vi "HandleObservationSync.vi"(8 "error in (no error)":errorcluster, 11 "S4GUI in":refnum<class "S4GUI.lvclass">) -> (0 "error out":errorcluster, 3 "S4GUI out":refnum<class "S4GUI.lvclass">)   [LabVIEW 2018, in "S4GUI.lvclass"] (continued)
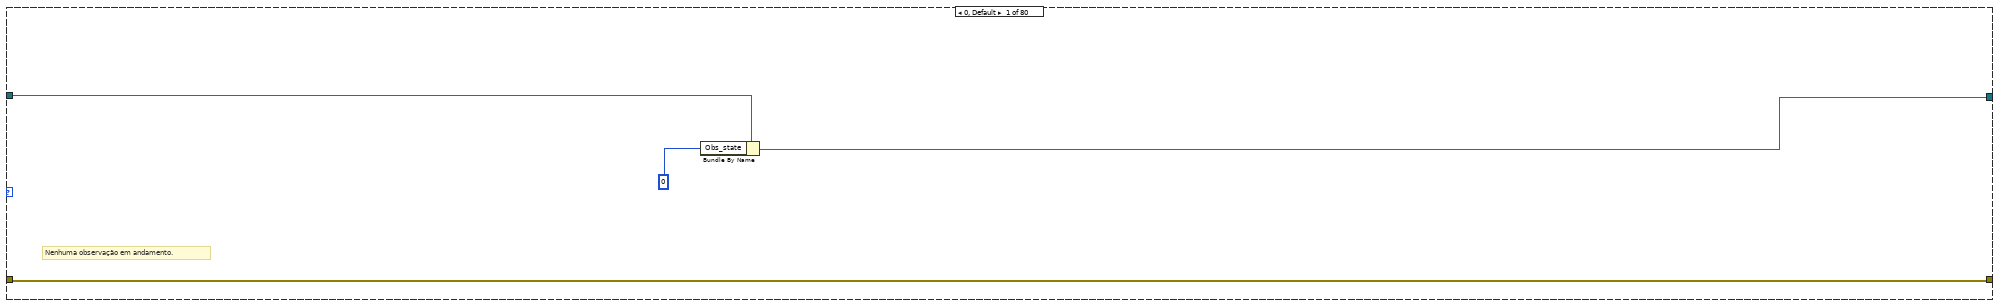
[diagram p2: hidden frame]
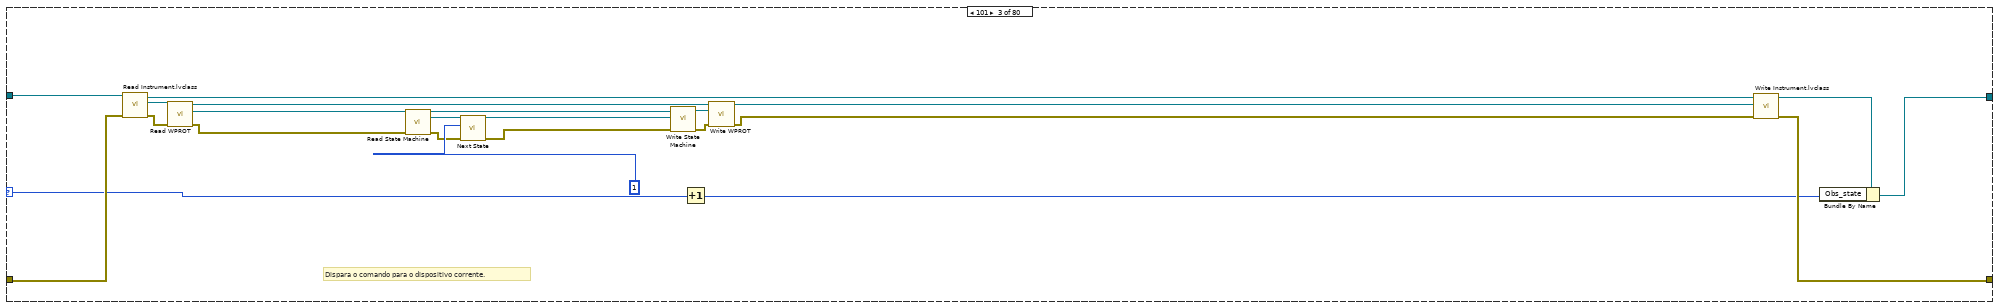
[diagram p4: hidden frame]
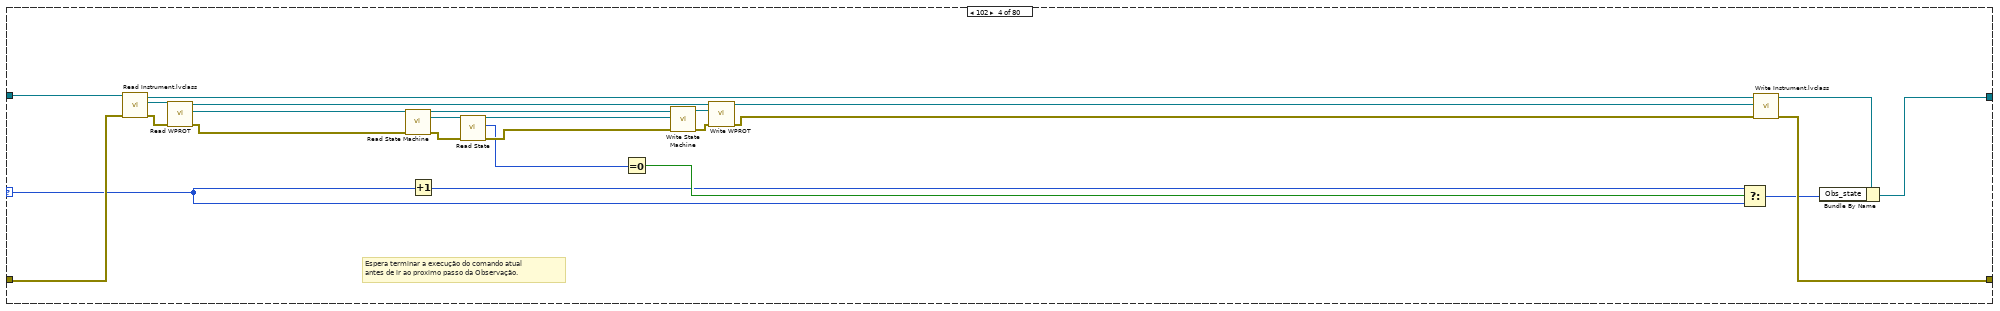
[diagram p5: hidden frame]
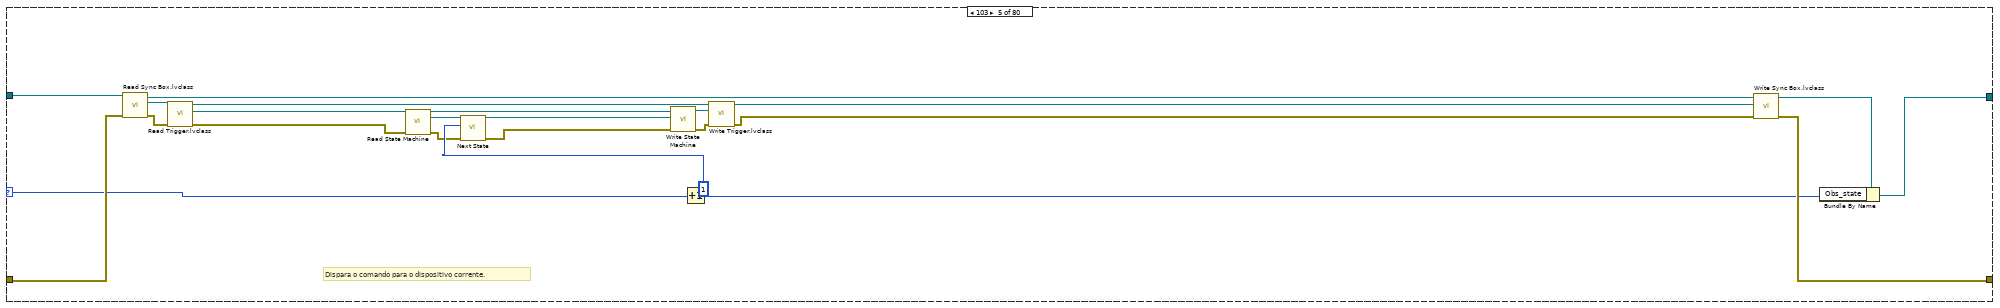
[diagram p6: hidden frame]
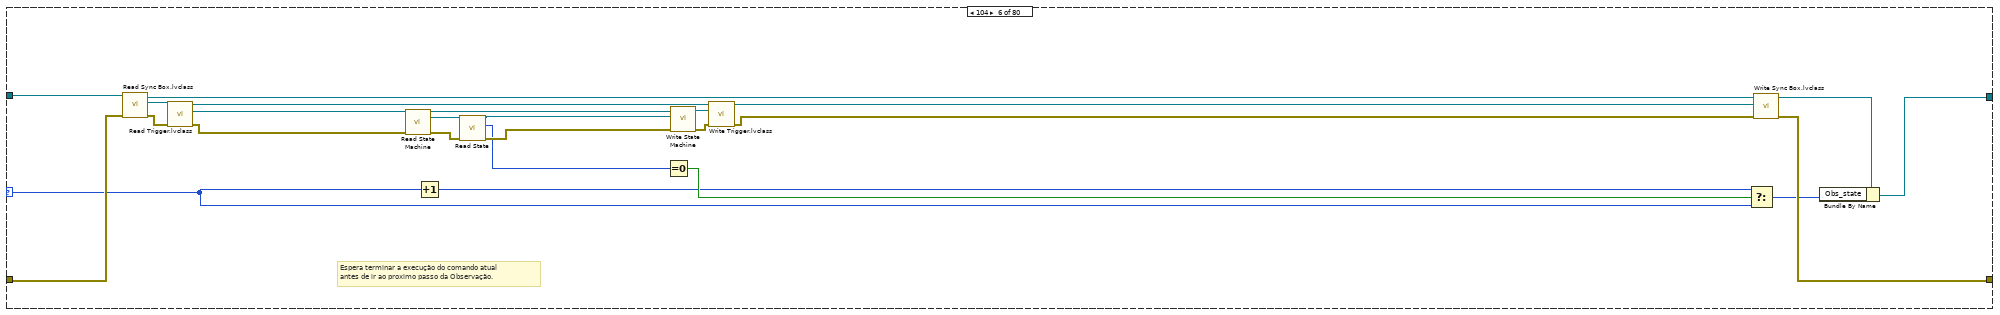
[diagram p7: hidden frame]
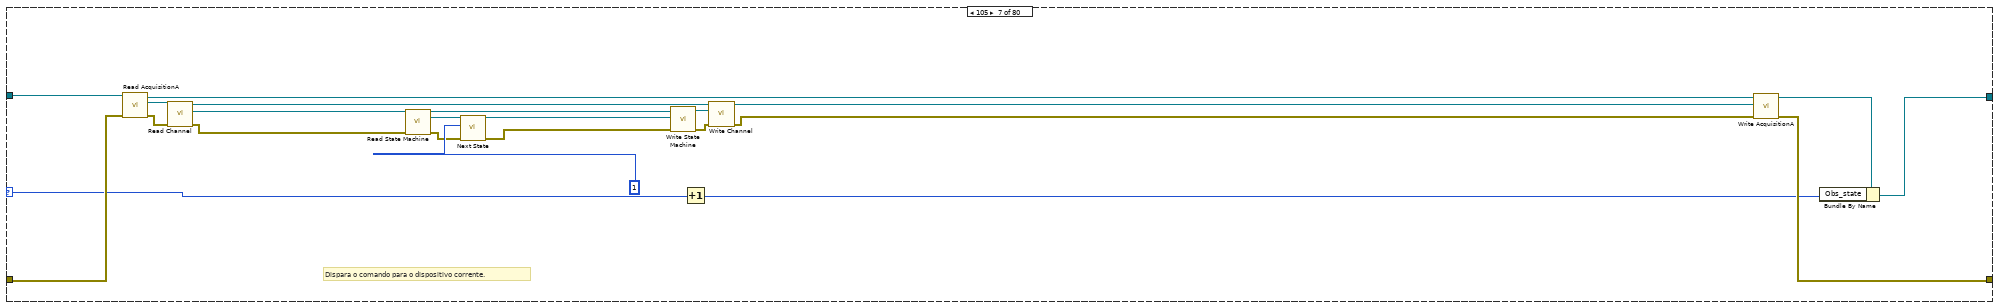
[diagram p8: hidden frame]
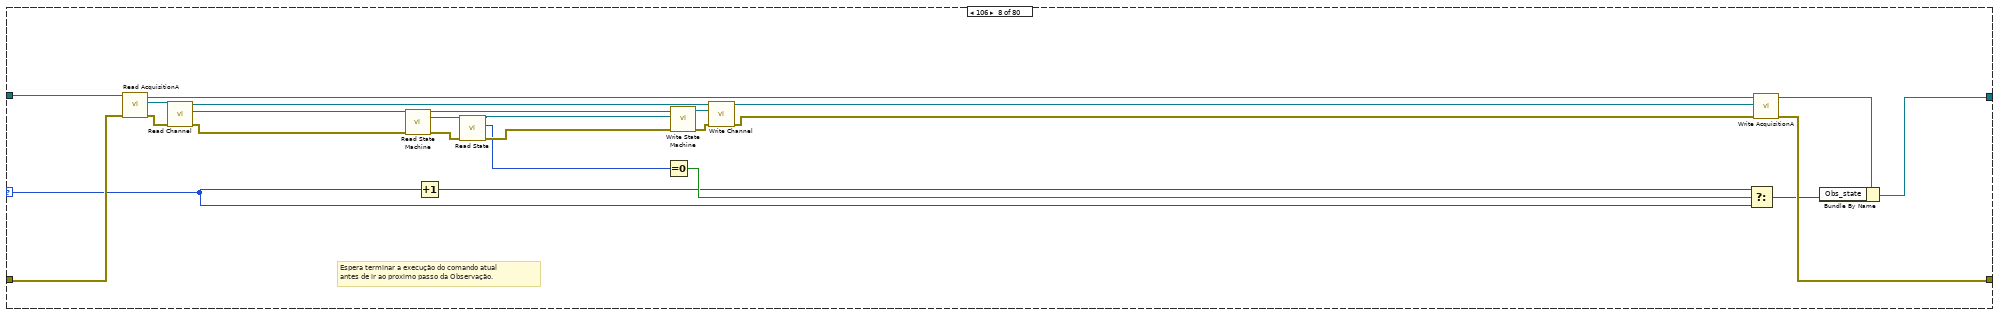
[diagram p9: hidden frame]
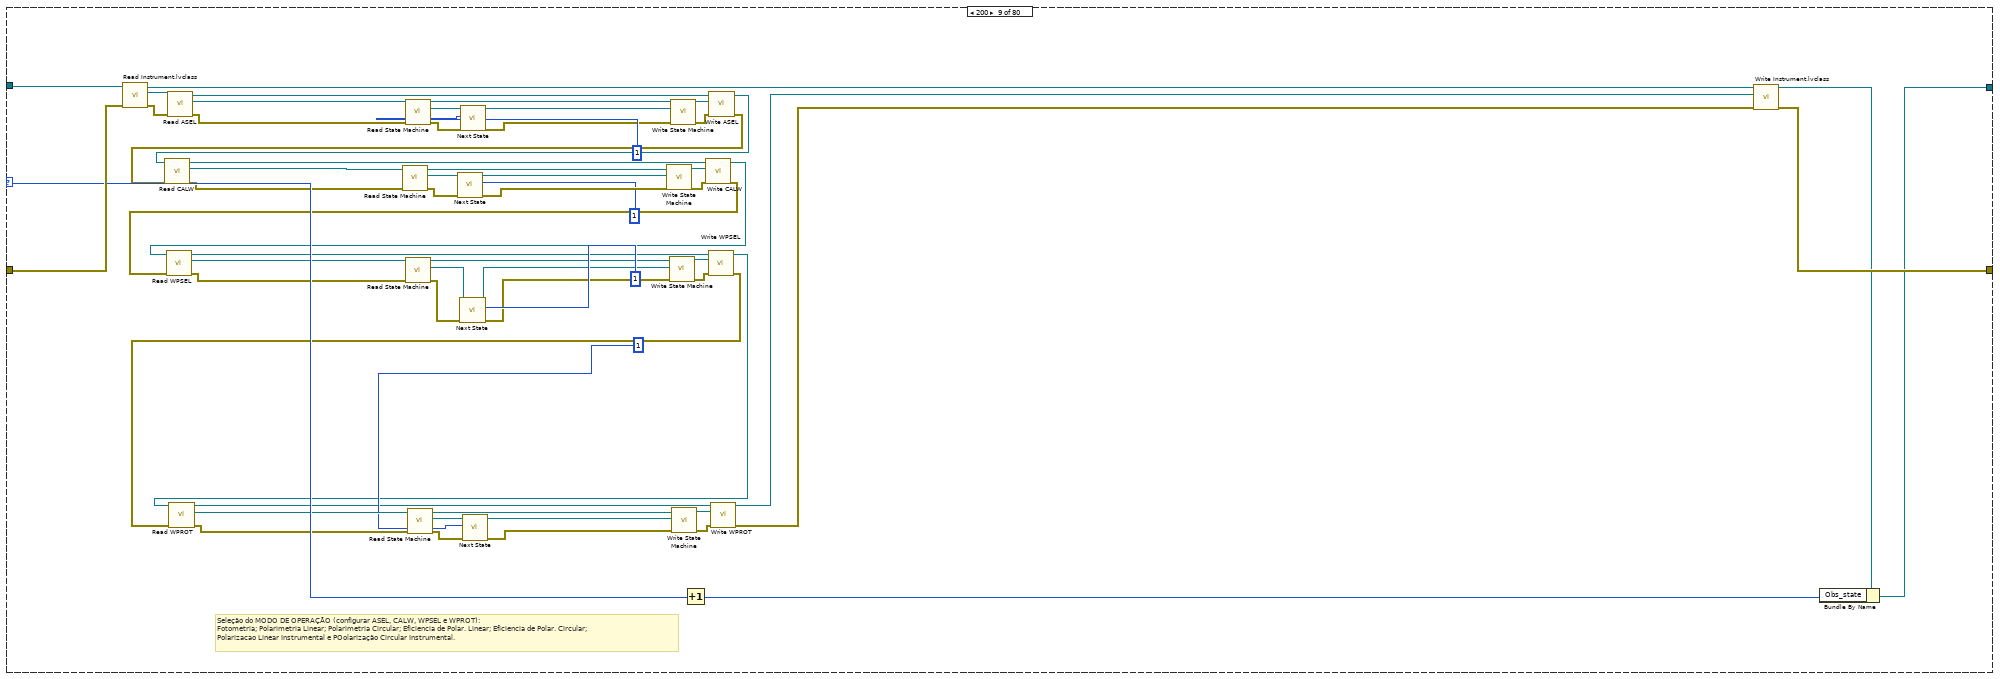
[diagram p10: hidden frame]
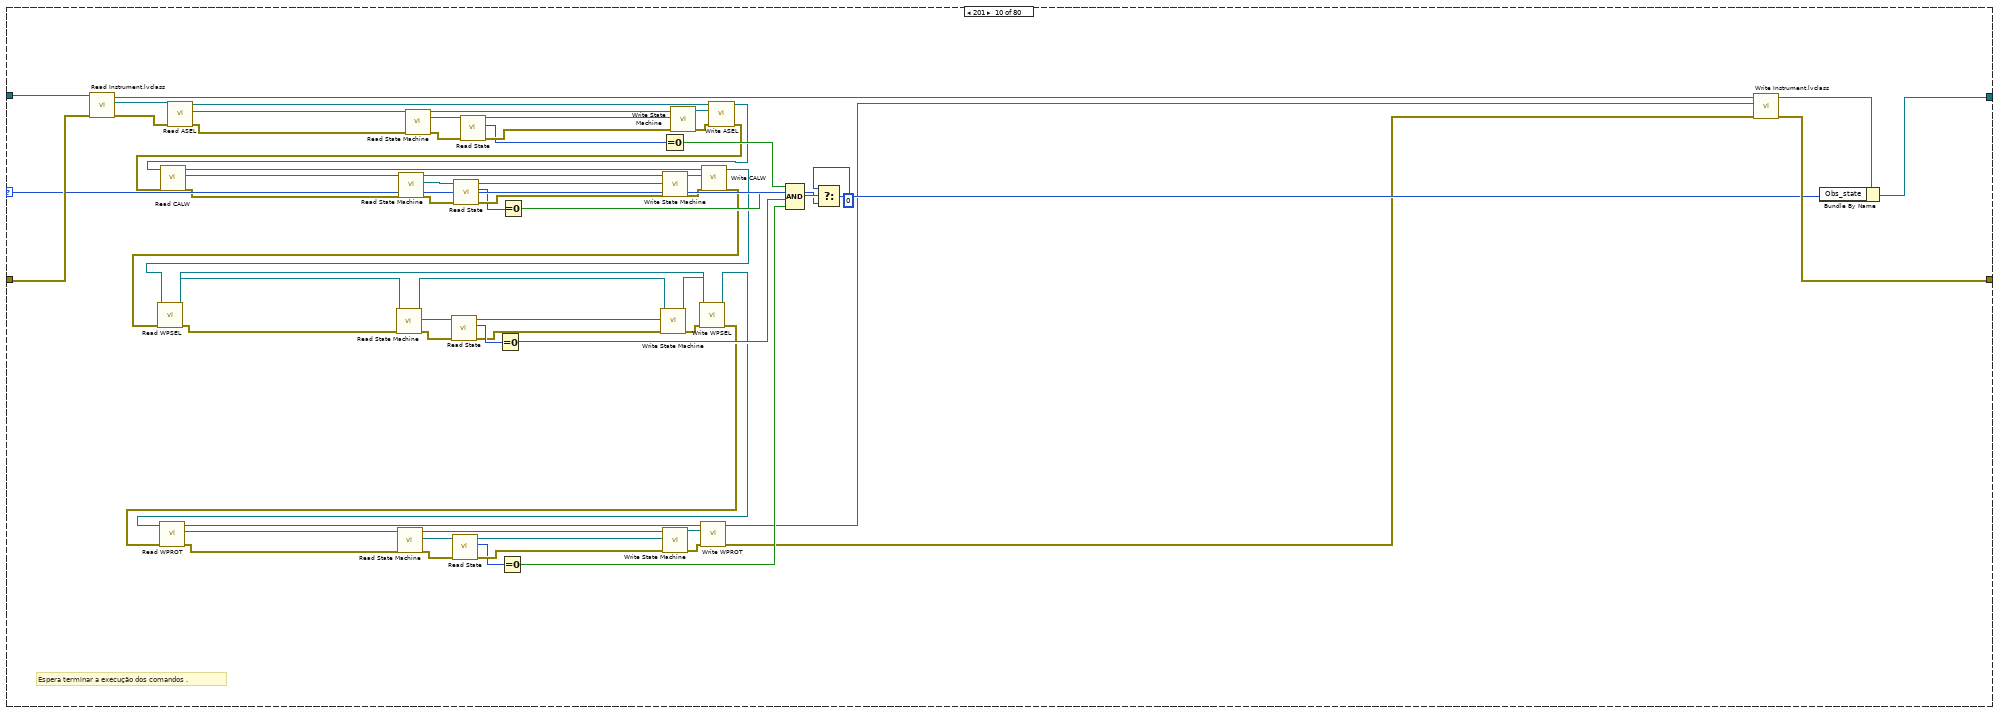
[diagram p11: hidden frame]
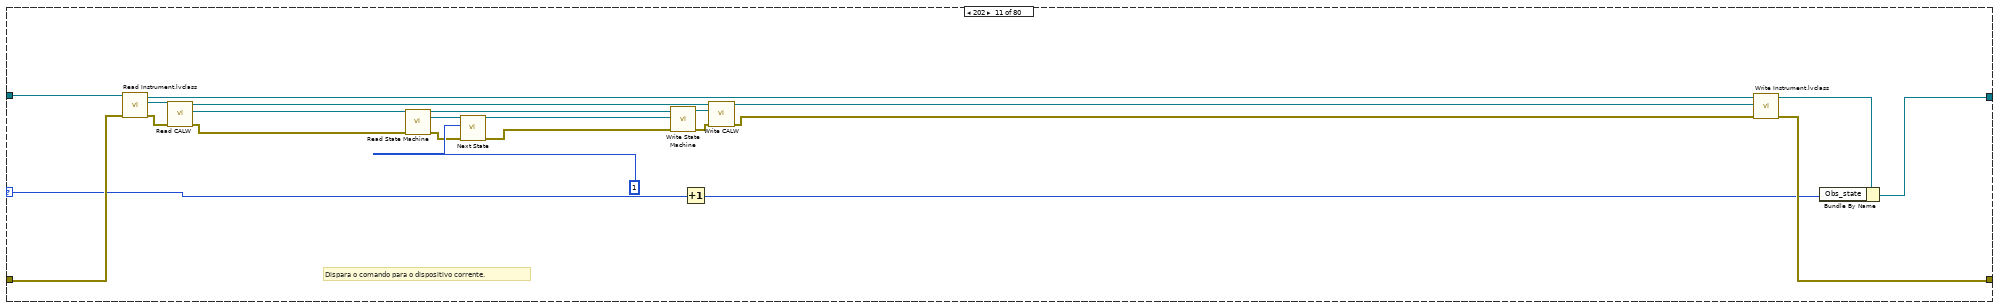
[diagram p12: hidden frame]
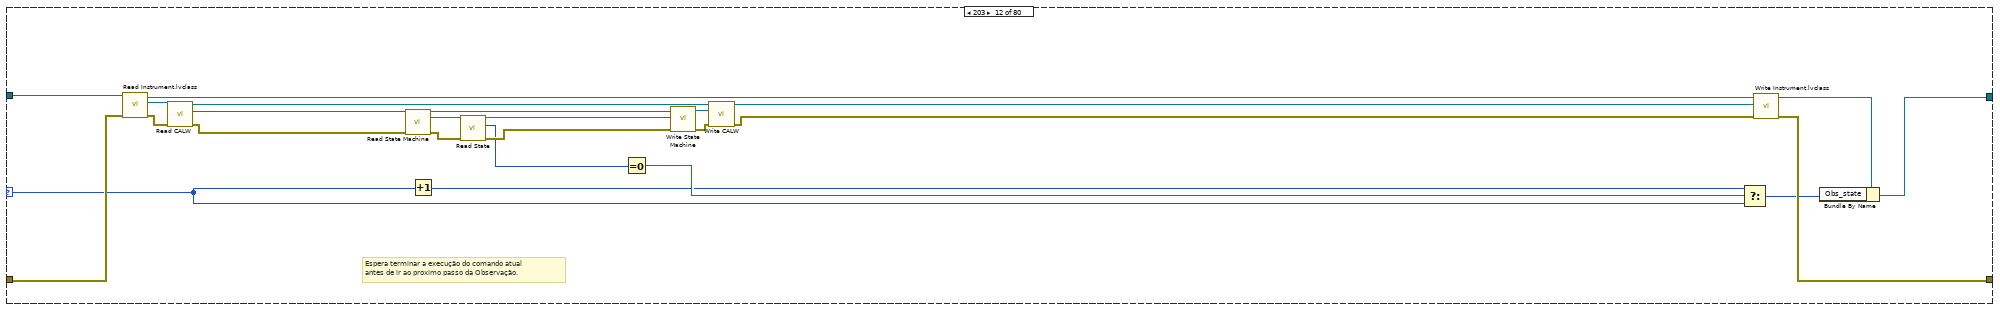
[diagram p13: hidden frame]
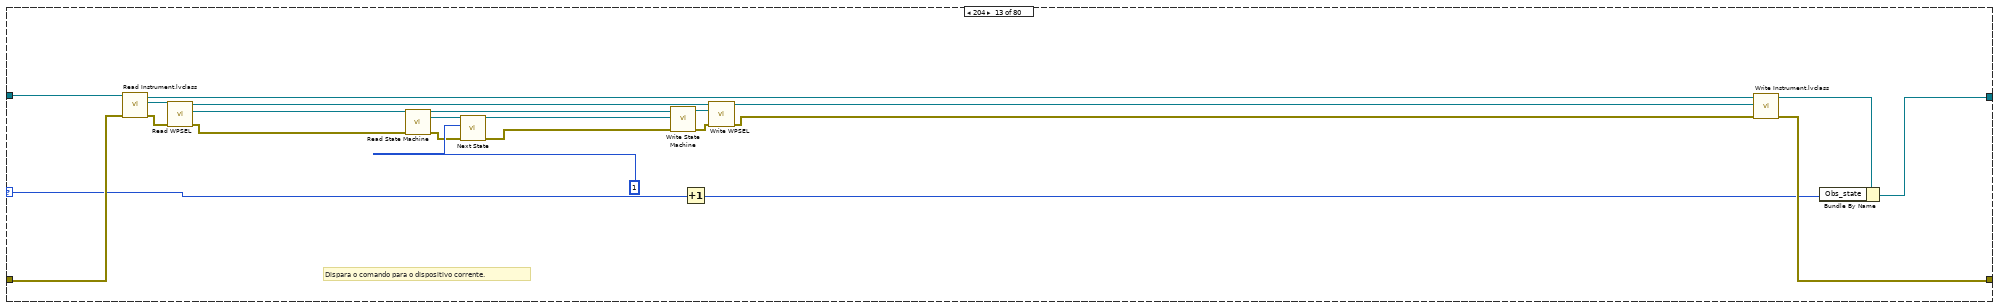
[diagram p14: hidden frame]
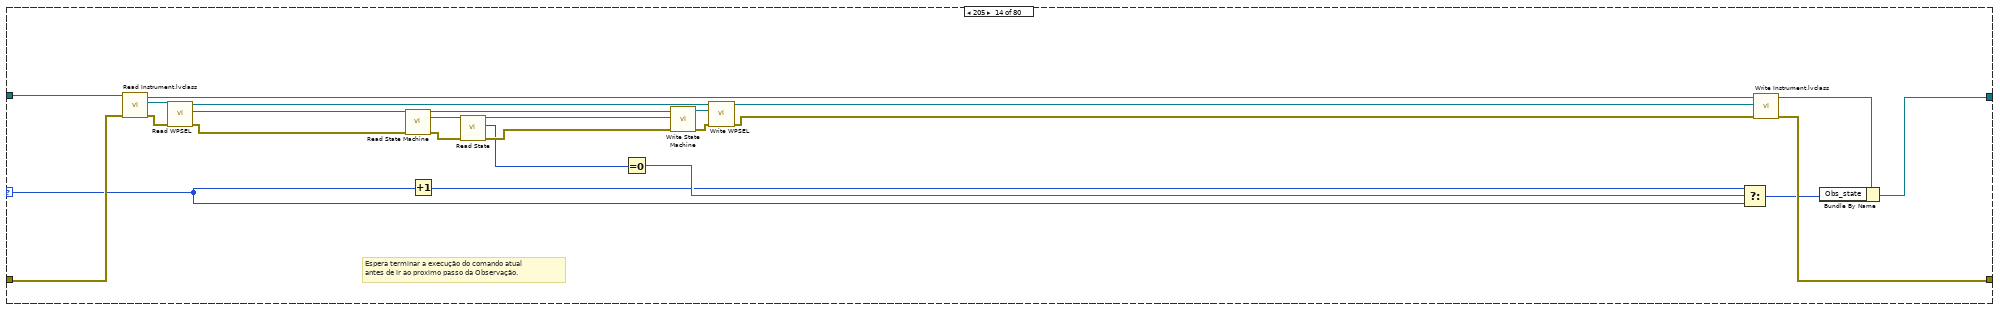
[diagram p15: hidden frame]
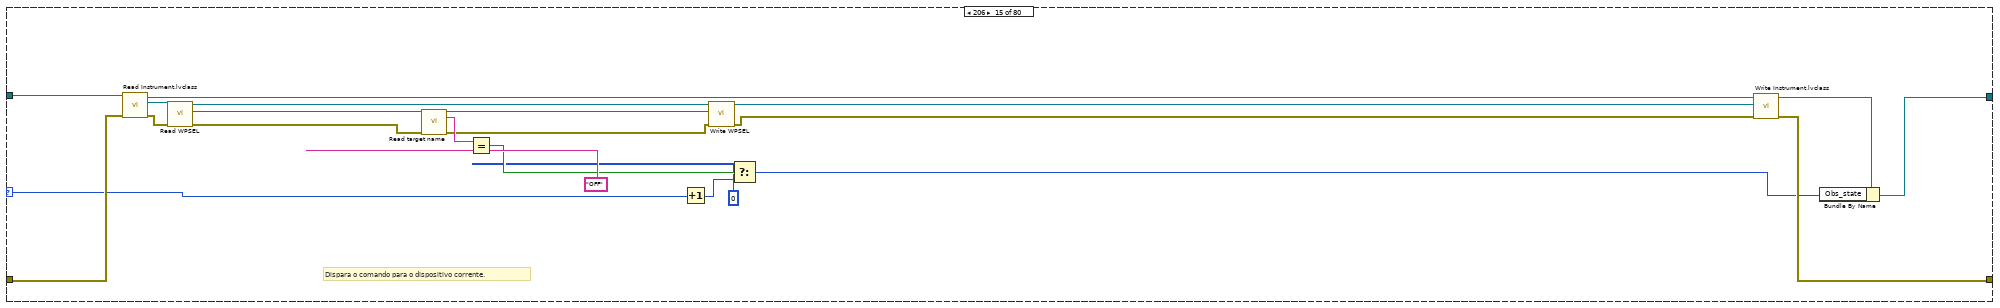
[diagram p16: hidden frame]
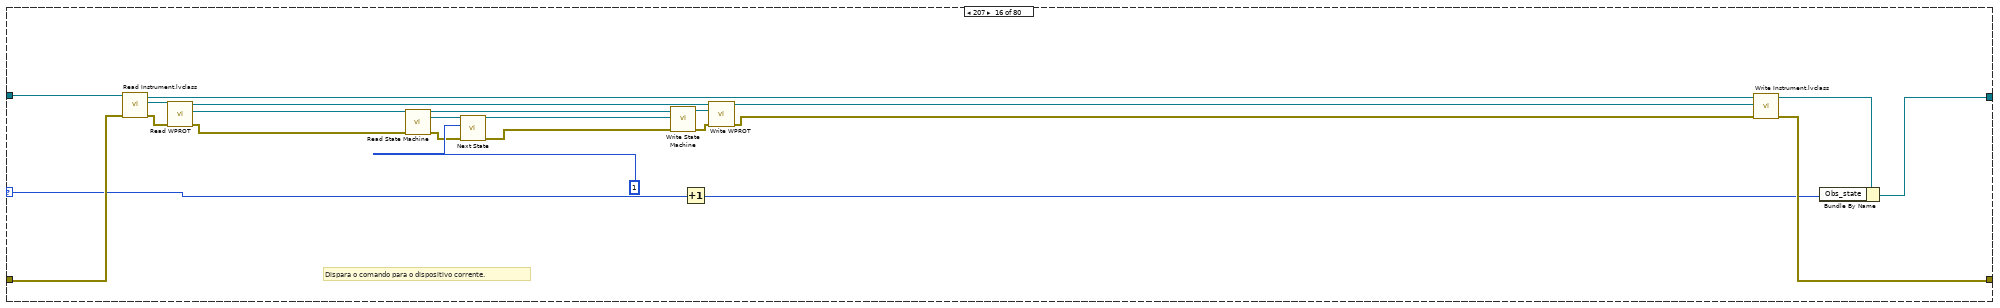
[diagram p17: hidden frame]
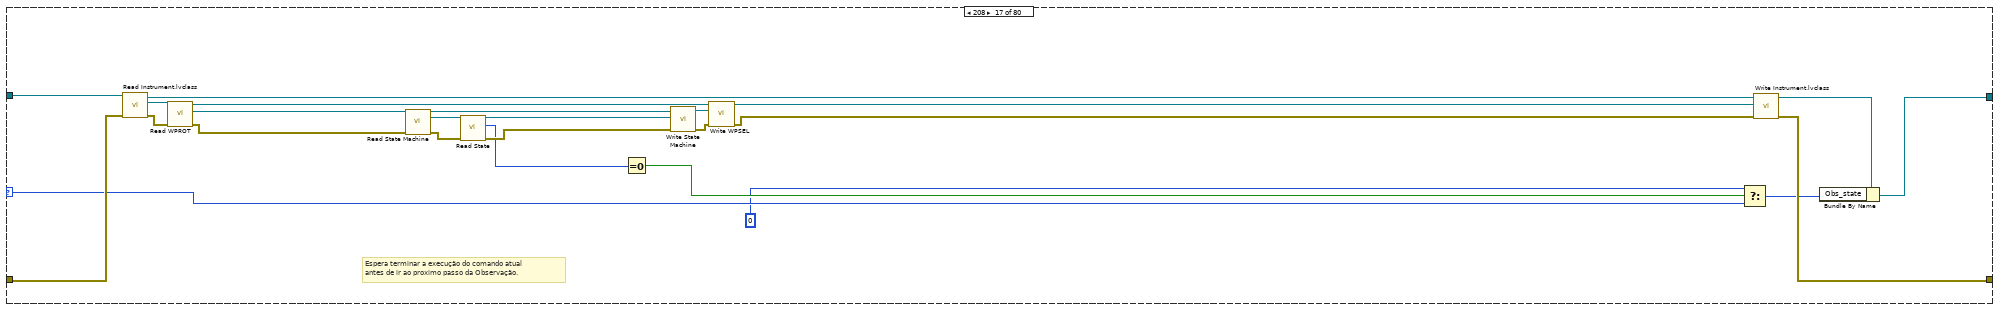
[diagram p18: hidden frame]
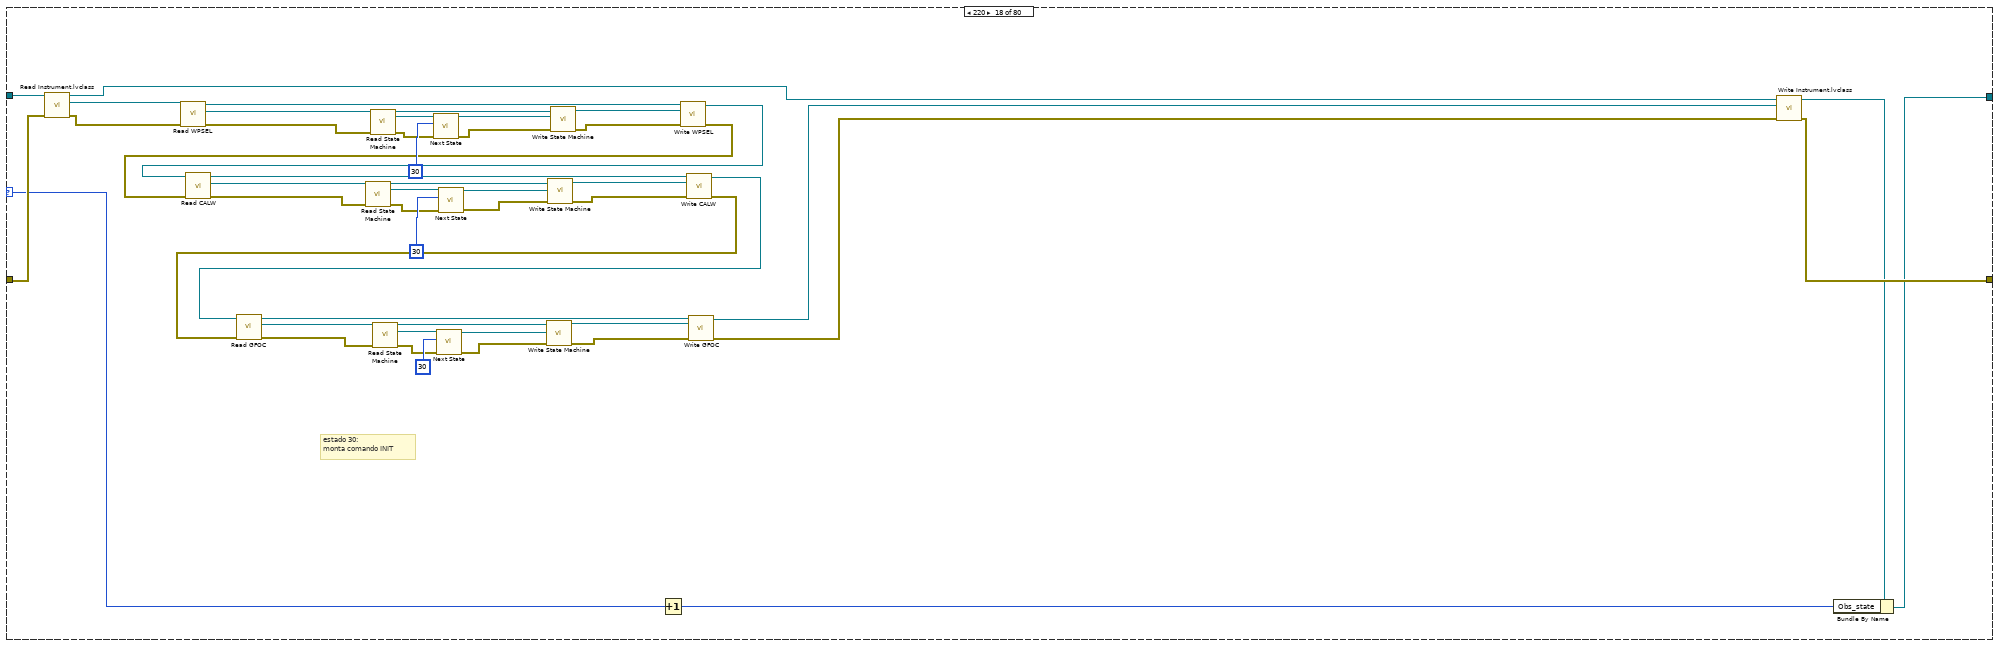
[diagram p19: hidden frame]
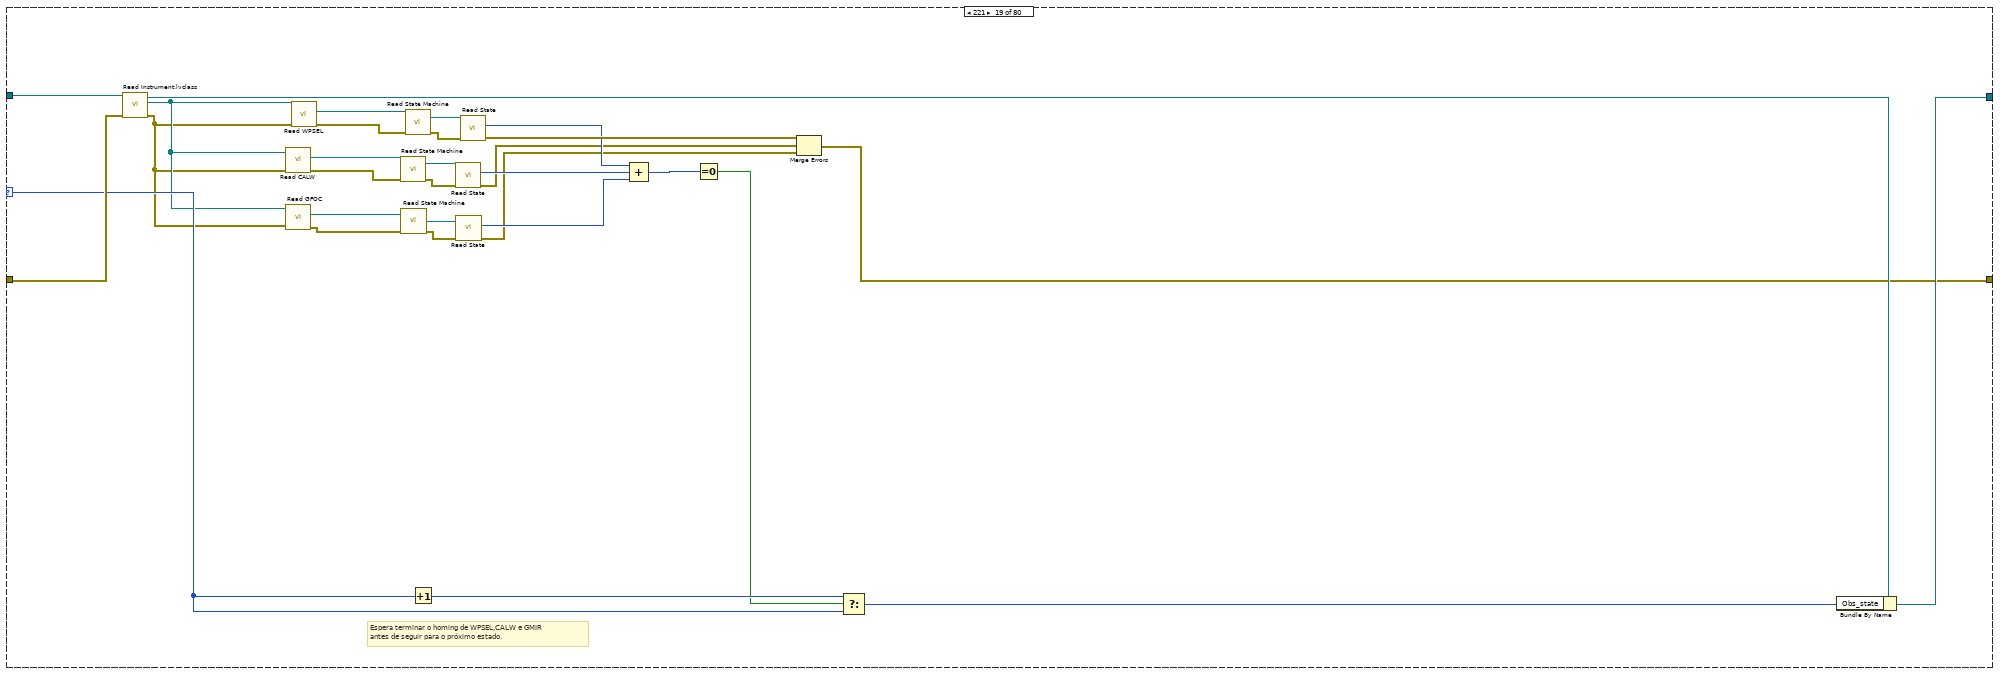
[diagram p20: hidden frame]
                      n2098 = Bundle By Name(cluster=w5788, "Obs_state"=w5785, "sequesDone"=w5784, "cyclesDone"=w5784) -> (w5787:refnum<class "S4GUI.lvclass">)
                    }
                  }
                }
              }
            }
          }
        }
        frame 368 {
          n2099 = Unbundle By Name(w5890) -> ("TelFocus.lvclass"=w5889:refnum<class "TelFocus.lvclass">)
          n2100 = call-dynamic "VerifSteps.vi"("error in (no error)"=w5886, "TelFocus in"=w5889) -> ("error out"=w5885:errorcluster, "continua?"=w5891:bool, "TelFocus out"=w5888:refnum<class "TelFocus.lvclass">)  [unwired: 7 in]
          n2101 = Bundle By Name(cluster=w5890, "TelFocus.lvclass"=w5888) -> (w5887:refnum<class "S4GUI.lvclass">)
          n2102 = Select(t=u32 360, s=w5891, f=u32 0) -> (s? t:f=w5894:u32)
          n2103 = Bundle By Name(cluster=w5887, "Obs_state"=w5894) -> (w5895:refnum<class "S4GUI.lvclass">)
        }
        frame 400 {
          # "Estado de \"Pause\": fica parado aqui até o botão START seja pressionado."
        }
        frame 500 {
          # "Espera terminar o envio de RESUME para todos os ACS."
          # "Estado de \"Pause\": fica parado aqui até o botão START seja pressionado."
          n2104 = call-dynamic "VerifyAcqIdle.vi"("error in (no error)"=w5900, "S4GUI in"=w5904) -> ("error out"=w5899:errorcluster, "idle"=w5903:bool, "S4GUI out"=w5902:refnum<class "S4GUI.lvclass">)  [unwired: 6 in, 1 out]
          n2105 = case shown="True" w5903 {
            tunnel: w5902 -> [w5906 w5916]
            tunnel: [w5906 w5908] -> w5901
            tunnel: w5899 -> [w5905 w5915]
            tunnel: [w5905 w5909] -> w5898
            frame False {
            }
            frame True {
              n2106 = call-dynamic "LoadPrevAcqRunState.vi"("error in (no error)"=w5915, "S4GUI in"=w5916) -> ("error out"=w5910:errorcluster, "S4GUI out"=w5911:refnum<class "S4GUI.lvclass">)  [unwired: 8 in]
              n2107 = Tick Count (ms)() -> (millisecond timer value=w5907:u32)
              n2108 = call-dynamic "Read Obs_prevstate.vi"("error in (no error)"=w5910, "S4ACS_GUI in"=w5911) -> ("error out"=w5914:errorcluster, "Obs_prevstate"=w5912:u32, "S4ACS_GUI out"=w5913:refnum<class "S4GUI.lvclass">)  [unwired: 7 in]
              n2109 = local write "time307"(w5907) -> ()
              n2110 = local write "time1"(w5907) -> ()
              n2111 = call-dynamic "Write Obs_state.vi"("error in (no error)"=w5914, "Obs_state"=w5912, "S4ACS_GUI in"=w5913) -> ("error out"=w5909:errorcluster, "S4ACS_GUI out"=w5908:refnum<class "S4GUI.lvclass">)  [unwired: 7 in]
            }
          }
        }
      }
    }
    frame Error {
    }
  }
  "error out" <- w3
  "S4GUI out" <- w2
